vi "sub_resample_and_FSKdemodulate.vi"(1 "FSK Init Parameters":T1, 2 "error in (no error)":errorcluster, 3 "packet_arr":cdb[][](array[numeric]), 4 "Rx IQ Sampling\nRate [s/sec]":dbl) -> (7 "Sync Found":bool, 8 "recovered complex waveform":T2[](array[typedef]) {"Y" format="%.3f"; "dt" format="%^.2e"; "t0" format="%.4f"}, 9 "error out":errorcluster, 10 "output bit stream":i8[][](array[numeric]))   [LabVIEW 2015]
uses:
  <vilib>/addons/Modulation/Analog/controls/Complex Data Waveform.ctl
  <vilib>/addons/Modulation/Analog/support/Validators/mod_Fractional Resample Validate.vi
  <vilib>/addons/Modulation/Analog/support/Validators/mod_Check Flush State.vi
  <vilib>/addons/Modulation/Analog/support/mod_FractionalResampler.vi
  <vilib>/addons/Modulation/Analog/support/mod_Integer Rate Interpolation.vi
  <vilib>/addons/Modulation/Analog/support/mod_Set Error Source.vi
  <vilib>/addons/Modulation/Analog/support/Validators/mod_Validate Complex Waveform.vi
  <vilib>/addons/Modulation/Analog/support/mod_PerformResampling.vi
  <vilib>/addons/Modulation/Analog/support/Validators/mod_WFErrorHandler.vi
  <vilib>/Utility/error.llb/Error Cluster From Error Code.vi
  <vilib>/addons/Modulation/Analog/support/mod_Resampling Factors.vi
  <vilib>/addons/Modulation/Analog/support/mod_ResamplingFilter.vi
  <vilib>/addons/Modulation/Analog/support/mod_Generate Integer Interpolation Filter.vi
  <vilib>/addons/Modulation/niAMT.lvlib
  <vilib>/addons/Modulation/niDMT.lvlib
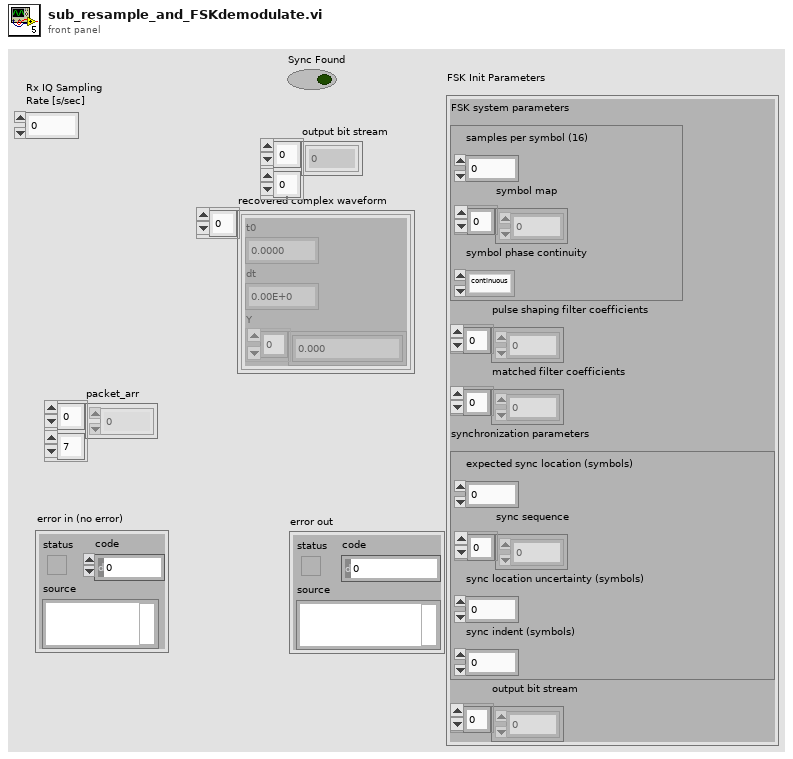
[diagram p1: front panel]
types:
  T1 = cluster{"FSK system parameters":cluster{"samples per symbol (16)":i32, "symbol map":dbl[], "symbol phase continuity":enum16{"continuous", "discontinuous"}}, "pulse shaping filter coefficients":dbl[], "matched filter coefficients":dbl[], "synchronization parameters":cluster{"expected sync location (symbols)":i32, "sync sequence":cdb[], "sync location uncertainty (symbols)":i32, "sync indent (symbols)":i32}, "output bit stream":i8[]}
  T2 = typedef "niAMT.lvlib/Complex Data Waveform.ctl" = cluster{"t0":dbl, "dt":dbl, "Y":cdb[]}
  T3 = cluster{"samples per symbol (16)":i32, "symbol map":dbl[], "symbol phase continuity":enum16{"continuous", "discontinuous"}}
  T4 = cluster{"expected sync location (symbols)":i32, "sync sequence":cdb[], "sync location uncertainty (symbols)":i32, "sync indent (symbols)":i32}
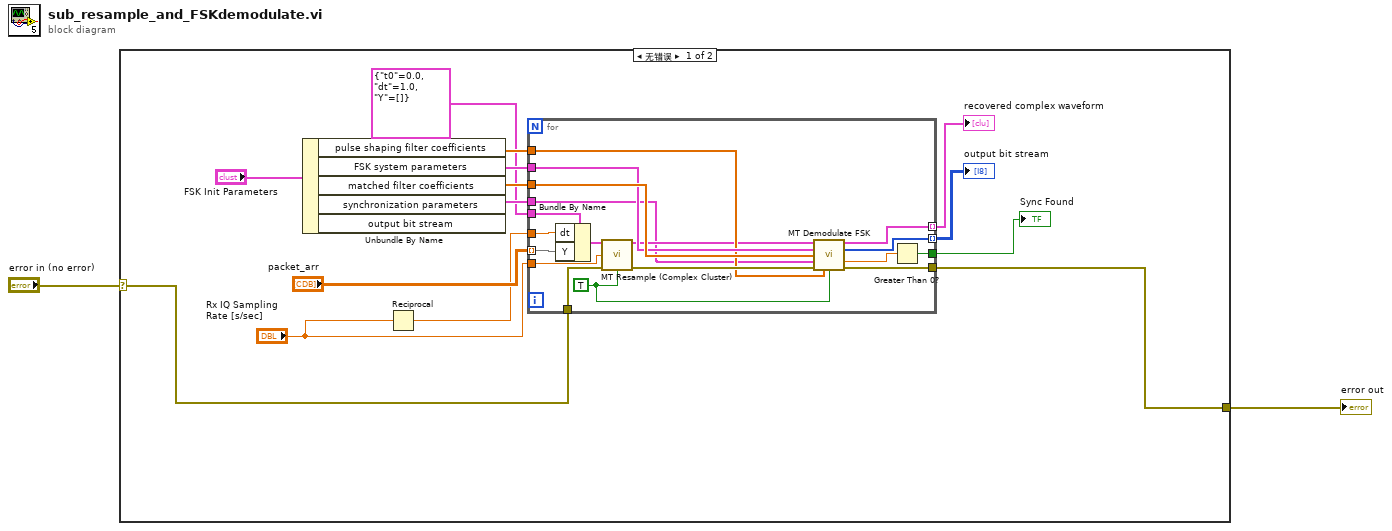
[diagram p0: block diagram]
diagram:
  n1 = case shown="无错误" "error in (no error)" {
    selector: "error in (no error)" -> [w5 w35]
    tunnel: [w14 w35] -> w2
    frame No Error {
      n2 = Unbundle By Name("FSK Init Parameters") -> ("pulse shaping filter coefficients"=w10:dbl[], "FSK system parameters"=w13:T3, "matched filter coefficients"=w12:dbl[], "synchronization parameters"=w11:T4)  [unwired: 1 out]
      n3 = Reciprocal(x="Rx IQ Sampling\nRate [s/sec]") -> (1/x=w7:dbl)
      n4 = for {
        tunnel: "packet_arr" -> [w22] mode=indexing
        tunnel: "Rx IQ Sampling\nRate [s/sec]" -> [w33]
        tunnel: w10 -> [w20]
        tunnel: w12 -> [w32]
        tunnel: w13 -> [w21]
        tunnel: [w31] -> w16 mode=indexing
        tunnel: w11 -> [w18]
        tunnel: [w30] -> w3
        tunnel: [w29] -> w14
        tunnel: [w27] -> w9 mode=indexing
        tunnel: w7 -> [w26]
        tunnel: T2 {"t0"=0.0, "dt"=1.0, "Y"=[]} ("input complex waveform") -> [w25]
        tunnel: w5 -> [w23]
        w28 = TRUE ("reset? (T)")
        n5 = Bundle By Name(cluster=w25, "dt"=w26, "Y"=w22) -> (w24:T2)
        n6 = call <vilib>:"MT Resample (Complex Cluster).vi"("input complex waveform"=w24, "desired sample rate (Hz)"=w33, "error in (no error)"=w23, "reset? (T)"=w28) -> ("output complex waveform"=w19:T2, "error out"=w34:errorcluster)  [unwired: 10 in]
        n7 = call <vilib>:"MT Demodulate FSK.vi"("input complex waveform"=w19, "FSK system parameters"=w21, "matched filter coefficients"=w32, "synchronization parameters"=w18, "error in (no error)"=w34, "pulse shaping filter coefficients"=w20, "reset? (T)"=w28) -> ("recovered complex waveform"=w27:T2, "output bit stream"=w31:i8[], "sync found index (symbols)"=w17:dbl, "error out"=w29:errorcluster)  [unwired: 4 in, 1 out]
        n8 = Greater Than 0?(x=w17) -> (x > 0?=w30:bool)
      }
      "Sync Found" <- w3
      "output bit stream" <- w16
      "recovered complex waveform" <- w9
    }
    frame Error {
    }
  }
  "error out" <- w2
